vi "Deliver Request.vi"(8 "error in (no error)":errorcluster, 10 "Request":refnum<class "request.lvclass">, 11 "output_poller_queue in":refnum<class "output_poller_queue.lvclass">) -> (0 "error out":errorcluster, 3 "output_poller_queue out":refnum<class "output_poller_queue.lvclass">)   [LabVIEW 2015, in "output_poller_queue.lvclass"]
uses:
  output_poller_queue.lvclass
  Request/request.lvclass
  output_poller_queue.lvclass/output_poller_queue.ctl
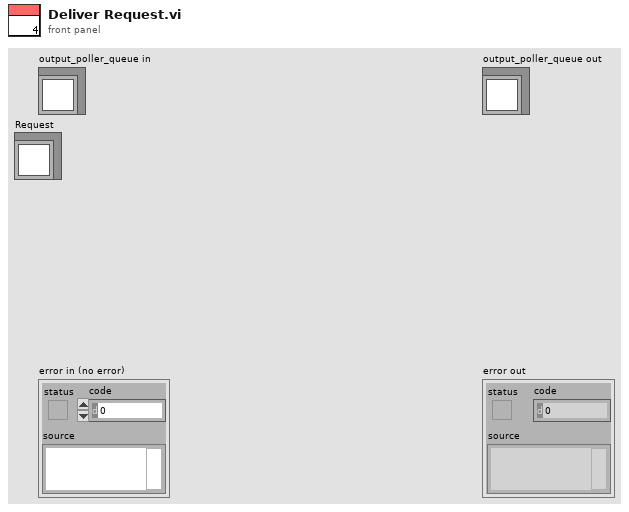
[diagram p1: front panel]
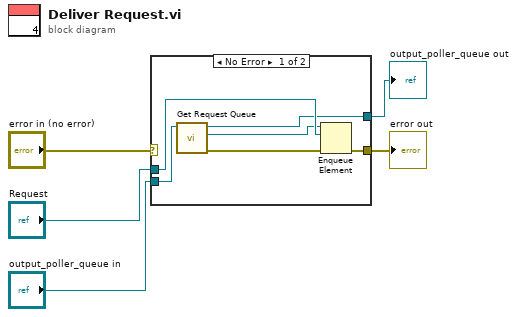
[diagram p0: block diagram]
diagram:
  n1 = case shown="No Error" "error in (no error)" {
    selector: "error in (no error)" -> [_ w13]
    tunnel: [w7 w13] -> w4
    tunnel: [w6 w12] -> w3
    tunnel: "output_poller_queue in" -> [w11 w12]
    tunnel: "Request" -> [w10 _]
    frame No Error {
      n2 = call "Get Request Queue.vi"("output_poller_queue in"=w11) -> ("error out"=w8:errorcluster, "request_queue"=w9:refnum<queue>, "output_poller_queue out"=w6:refnum<class "output_poller_queue.lvclass">)  [unwired: 8 in]
      n3 = Enqueue Element(queue=w9, element=w10, error in (no error)=w8) -> (error out=w7:errorcluster)  [unwired: 1 in, 2 out]
    }
    frame Error {
    }
  }
  "error out" <- w4
  "output_poller_queue out" <- w3
